vi "ParamClusterControl.vi"(9 "IO queue in":refnum<queue>, 10 "SetGetCommands":string="\n", 11 "Cluster ref":refnum<vi>) -> (1 "IO queue out":refnum<queue>, 3 "Command queue":refnum<queue>)   [LabVIEW 2021]
panel:
  # "呼び出し元 → Core\nコマンドを送るための Queue"
  # "書き込みコマンド\n読み出しコマンド\nScan フォーマット\nの3行を項目数分繰り返す"
  # "Core → 呼び出し元\nGetSetCommands に指定した\nコマンドが送られる Queue"
  # "指定しなければ内部で作成する\n指定すればそれを使う"
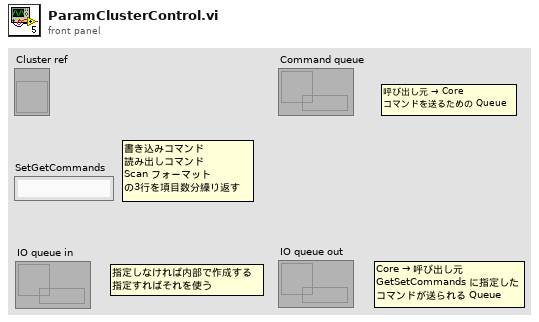
[diagram p1: front panel]
types:
  T1 = cluster{"Operation":enum16{"read", "write"}, "Data":string, "Queue":refnum<queue>}
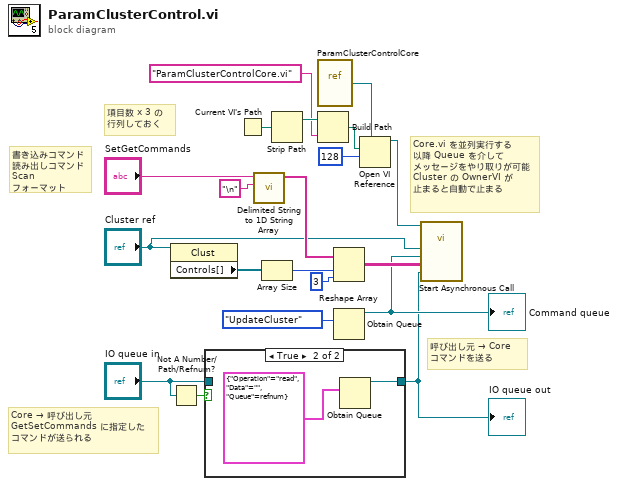
[diagram p0: block diagram]
diagram:
  # "呼び出し元 → Core\nコマンドを送る"
  # "Core → 呼び出し元\nGetSetCommands に指定した\nコマンドが送られる"
  # "Core.vi を並列実行する\n以降 Queue を介して\nメッセージをやり取りが可能\nCluster の OwnerVI が\n止まると自動で止まる"
  # "項目数 x 3 の\n行列しておく"
  # "書き込みコマンド\n読み出しコマンド\nScan フォーマット"
  n1 = property class="Clust"(reference="Cluster ref") -> ("Controls[]"=w14:refnum<vi>[])  [unwired: 1 in, 2 out]
  n2 = Not A Number/Path/Refnum?(number/path/refnum="IO queue in") -> (NaN/Path/Refnum?=w3:bool)
  n3 = case shown="True" w3 {
    tunnel: "IO queue in" -> [w21 _]
    tunnel: [w21 w22] -> w1
    frame False {
    }
    frame True {
      n4 = Obtain Queue(element data type=T1 {"Operation"=enum."read", "Data"="", "Queue"=refnum} ("IO Queue Packet (dummy)")) -> (queue out=w22:refnum<queue>)  [unwired: 4 in, 2 out]
    }
  }
  "IO queue out" <- w1
  n5 = Current VI's Path() -> (path=w12:path)
  n6 = call <vilib>:"Delimited String to 1D String Array.vi"("delimiter"="\n", "delimited string"="SetGetCommands") -> ("string array"=w18:string[])  [unwired: 9 in]
  n7 = Array Size(array=w14) -> (size(s)=w17:i32)
  n8 = Strip Path(path=w12) -> (stripped path=w11:path)  [unwired: 1 out]
  n9 = vi-ref "ParamClusterControlCore.vi"() -> (w13:refnum<vi>)
  n10 = Build Path(base path=w11, name or relative path="ParamClusterControlCore.vi") -> (appended path=w9:path)
  n11 = Reshape Array(w18, w17, 3 ("dimension size")) -> (w15:string[][])
  n12 = Obtain Queue(element data type=enum16{"UpdateCluster", "ClusterChanged"}."UpdateCluster") -> (queue out=w4:refnum<queue>)  [unwired: 4 in, 2 out]
  "Command queue" <- w4
  n13 = Open VI Reference(type specifier VI Refnum (for type only)=w13, vi path=w9, options=128) -> (vi reference=w8:refnum<vi>)  [unwired: 3 in, 1 out]
  n14 = call-by-ref "Start Asynchronous Call"(reference=w8, "IO queue"=w1, "SetGetCommands"=w15, "Command queue"=w4, "Cluster ref"="Cluster ref") -> ()  [unwired: 9 in, 2 out]
